vi "string to number formatted.vi"(7 "format string":string, 11 "Numeric":dbl) -> (3 "number string":string)   [LabVIEW 2025]
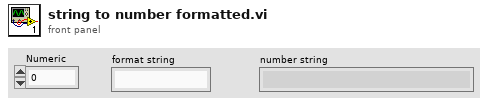
[diagram p1: front panel]
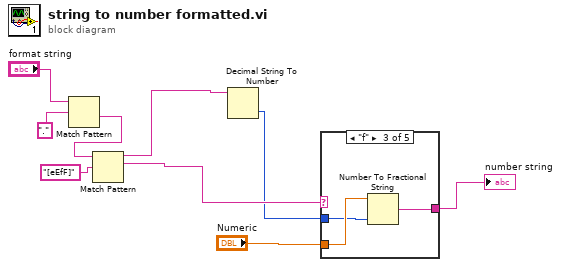
[diagram p0: block diagram]
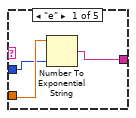
[diagram p2: hidden frame]
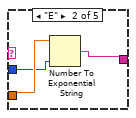
[diagram p3: hidden frame]
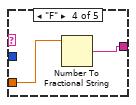
[diagram p4: hidden frame]
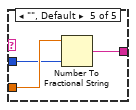
[diagram p5: hidden frame]
diagram:
  n1 = Match Pattern(string="format string", regular expression=".") -> (after substring=w6:string)  [unwired: 1 in, 3 out]
  n2 = Match Pattern(string=w6, regular expression="[eEfF]") -> (before substring=w3:string, match substring=w8:string)  [unwired: 1 in, 2 out]
  n3 = Decimal String To Number(string=w3) -> (number=w4:i32)  [unwired: 2 in, 1 out]
  n4 = case shown="\"f\"" w8 {
    tunnel: "Numeric" -> [w11 w15 w18 w20 w23]
    tunnel: [w12 w14 w17 w19 w22] -> w7
    tunnel: w4 -> [w10 w13 w16 _ w21]
    frame "e" {
      n5 = Number To Exponential String(number=w11, precision (6)=w10) -> (E-format string=w12:string)  [unwired: 2 in]
    }
    frame "E" {
      n6 = Number To Exponential String(number=w15, precision (6)=w13) -> (E-format string=w14:string)  [unwired: 2 in]
    }
    frame "f" {
      n7 = Number To Fractional String(number=w18, precision (6)=w16) -> (F-format string=w17:string)  [unwired: 2 in]
    }
    frame "F" {
      n8 = Number To Fractional String(number=w20) -> (F-format string=w19:string)  [unwired: 3 in]
    }
    frame "", Default {
      n9 = Number To Fractional String(number=w23, precision (6)=w21) -> (F-format string=w22:string)  [unwired: 2 in]
    }
  }
  "number string" <- w7
